vi "TimerForAndorSubvi.vi"(9 "y":dbl=15.0, 10 "period":dbl=20.0 format="%#_13g", 11 "milliseconds to wait":u32=1000) -> ()   [LabVIEW 2017]
uses:
  <vilib>/DAQmx/write.llb/DAQmx Write (Digital Bool 1Line 1Point).vi
  <vilib>/DAQmx/create/channels.llb/DAQmx Create Channel (DO-Digital Output).vi
  <vilib>/DAQmx/miscellaneous.llb/DAQmx Fill In Error Info.vi
panel:
  out "floor(x/y) 2":i32
  out "floor(x/y)":dbl=15.0
  out "x >= y?":bool=TRUE
  out "Numeric":i32=35
  in  "stop 3":bool
  out "error out":errorcluster
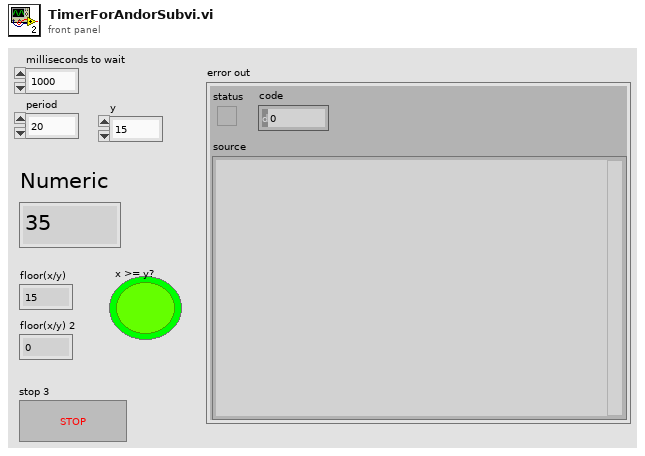
[diagram p1: front panel]
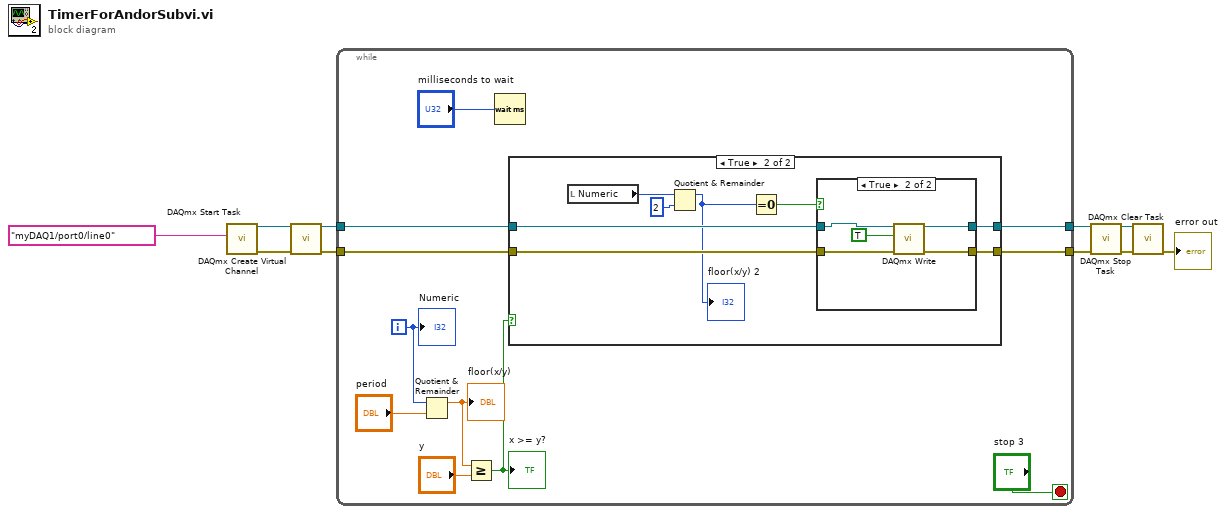
[diagram p0: block diagram]
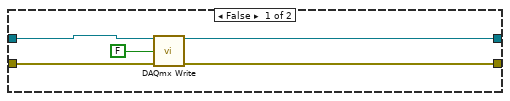
[diagram p2: hidden frame]
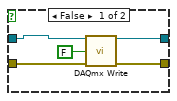
[diagram p3: hidden frame]
diagram:
  n1 = call-poly <vilib>:"DAQmx Create Virtual Channel.vi"("lines"=tag "myDAQ1/port0/line0") -> ("task out"=w10:refnum<k21>, "error out"=w8:errorcluster)  [unwired: 13 in]
  n2 = call <vilib>:"DAQmx Start Task.vi"("task/channels in"=w10, "error in"=w8) -> ("task out"=w5:refnum<k21>, "error out"=w4:errorcluster)  [unwired: 12 in]
  n3 = while {
    tunnel: w5 -> [w20]
    tunnel: w4 -> [w19]
    tunnel: [w18] -> w3
    tunnel: [w17] -> w2
    i -> [w15]
    stop <- "stop 3" stop-if-true
    n4 = Quotient & Remainder(x=w15, y="period") -> (x-y*floor(x/y)=w12:dbl)  [unwired: 1 out]
    "floor(x/y)" <- w12
    n5 = Greater Or Equal?(x=w12, y="y") -> (x >= y?=w11:bool)
    "x >= y?" <- w11
    n6 = Wait (ms)(milliseconds to wait="milliseconds to wait") -> ()  [unwired: 1 out]
    n7 = case shown="True" w11 {
      tunnel: w20 -> [w26 w34]
      tunnel: w19 -> [w25 w32]
      tunnel: [w24 w33] -> w18
      tunnel: [w23 w31] -> w17
      frame False {
        n8 = call-poly <vilib>:"DAQmx Write.vi"("task/channels in"=w26, "data"=FALSE, "error in"=w25) -> ("task out"=w24:refnum<k21>, "error out"=w23:errorcluster)  [unwired: 10 in, 1 out]
      }
      frame True {
        n9 = local read "Numeric"() -> (w30:i32)
        n10 = Quotient & Remainder(x=w30, y=2) -> (x-y*floor(x/y)=w27:i32)  [unwired: 1 out]
        "floor(x/y) 2" <- w27
        n11 = Equal To 0?(x=w27) -> (x = 0?=w29:bool)
        n12 = case shown="True" w29 {
          tunnel: w34 -> [w39 w44]
          tunnel: [w38 w43] -> w33
          tunnel: w32 -> [w37 w42]
          tunnel: [w36 w41] -> w31
          frame False {
            n13 = call-poly <vilib>:"DAQmx Write.vi"("task/channels in"=w39, "data"=FALSE, "error in"=w37) -> ("task out"=w38:refnum<k21>, "error out"=w36:errorcluster)  [unwired: 10 in, 1 out]
          }
          frame True {
            n14 = call-poly <vilib>:"DAQmx Write.vi"("task/channels in"=w44, "data"=TRUE, "error in"=w42) -> ("task out"=w43:refnum<k21>, "error out"=w41:errorcluster)  [unwired: 10 in, 1 out]
          }
        }
      }
    }
    "Numeric" <- w15
  }
  n15 = call <vilib>:"DAQmx Stop Task.vi"("task/channels in"=w3, "error in"=w2) -> ("task out"=w9:refnum<k21>, "error out"=w7:errorcluster)  [unwired: 12 in]
  n16 = call <vilib>:"DAQmx Clear Task.vi"("task in"=w9, "error in"=w7) -> ("error out"=→"error out":errorcluster)  [unwired: 13 in]
